vi "AH Bridge Parameters.vi"(0 "Instruments":T1[](array[typedef]), 5 "NML Addresses":string[](array[string]), 7 "Parameters":variant, 9 "Address":u16(ring) items=["GPIB 0 - Address 11", "GPIB 0 - Address 14"]) -> (1 "Show Firmware Warning":bool, 2 "Setting":u32, 3 "Model":string, 4 "VISA Resource Name":refnum<visa-resource-name>, 6 "Minimum":dbl, 8 "Is AH 2500":bool, 10 "Averaging Time":string[](array[string]), 12 "NML Addresses":string[](array[string]), 13 "Title":string, 14 "Wait Time (mS)":u32, 15 "Frequency":dbl)   [LabVIEW 2020]
uses:
  Sub Controls/Instrument Match.ctl
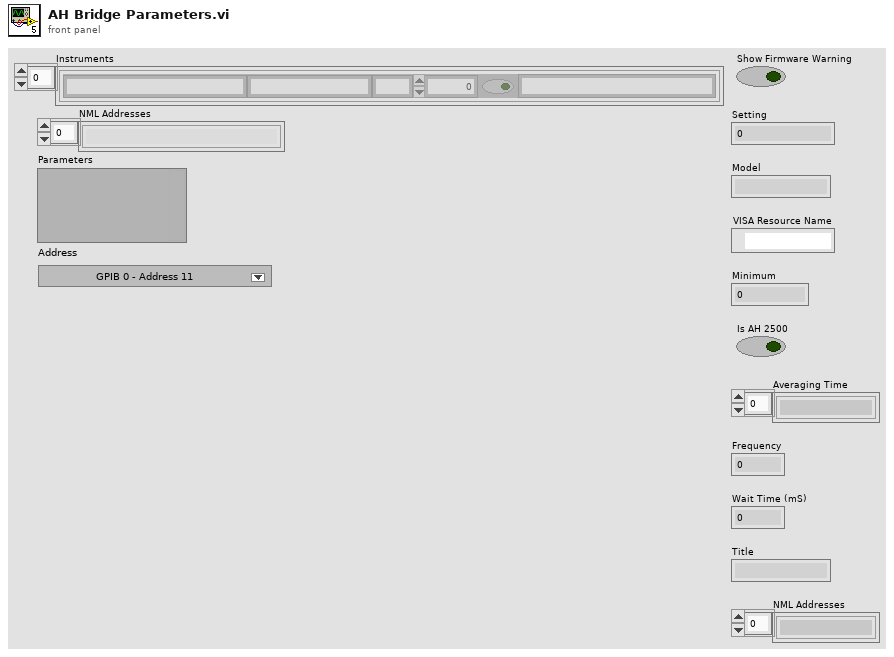
[diagram p1: front panel]
types:
  T1 = typedef "Instrument Match.ctl" = cluster{"Model":string, "Manufacturer":string, "Term Character":string, "Wait Time (mS)":u32, "Wait for SRQ":bool, "Type":string}
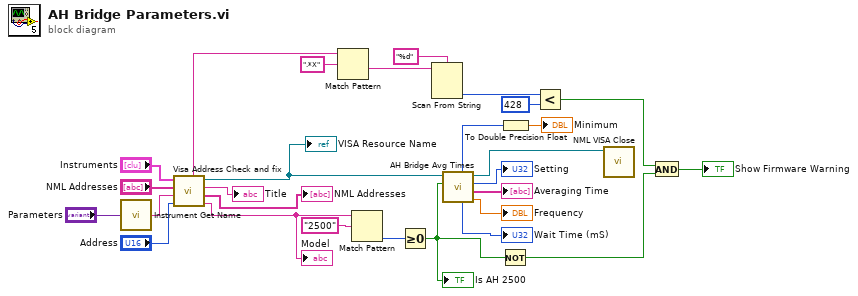
[diagram p0: block diagram]
diagram:
  n1 = call "Instrument Get Name.vi"("Parameters"="Parameters") -> ("Type"=w4:string)
  n2 = call "Visa Address Check and fix.vi"("Address"="Address", "Name"=w4, "NML Addresses"="NML Addresses", "Instruments"="Instruments") -> ("Model"=w26:string, "NML Addresses"=→"NML Addresses":string[], "Title"=→"Title":string, "VISA resource name"=w2:refnum<visa-resource-name>, "Firmware"=w17:string)  [unwired: 1 out]
  "Model" <- w26
  "VISA Resource Name" <- w2
  n3 = Match Pattern(string=w17, regular expression=".*X") -> (after substring=w16:string)  [unwired: 1 in, 3 out]
  n4 = Match Pattern(string=w26, regular expression="2500") -> (offset past match=w6:i32)  [unwired: 1 in, 3 out]
  n5 = Greater Or Equal To 0?(x=w6) -> (x >= 0?=w22:bool)
  "Is AH 2500" <- w22
  n6 = Scan From String(format string="%d", input string=w16) -> (output 1=w18:i32)  [unwired: 3 in, 3 out]
  n7 = call "AH Bridge Avg Times.vi"("VISA Resource name"=w2, "Is model 2500?"=w22) -> ("Min Setting"=w24:u32, "Wait Time (mS)"=→"Wait Time (mS)":u32, "VISA Resource out"=w1:refnum<visa-resource-name>, "Setting"=→"Setting":u32, "Averaging Time"=→"Averaging Time":string[], "Frequency"=→"Frequency":dbl)  [unwired: 2 in]
  n8 = Not(x=w22) -> (.not. x?=w23:bool)
  n9 = To Double Precision Float(number=w24) -> (double precision float=→"Minimum":dbl)
  n10 = Less?(x=w18, y=428) -> (x < y?=w20:bool)
  n11 = call "NML VISA Close.vi"("VISA resource name"=w1) -> ()  [unwired: 10 in, 1 out]
  n12 = And(x=w20, y=w23) -> (x .and. y?=→"Show Firmware Warning":bool)
